vi "buildquery.vi"(1 "String":string="status") -> (0 "JSON字符串":string)   [LabVIEW 2017]
panel:
  in  "输入簇":cluster{"command":string, "item":string}
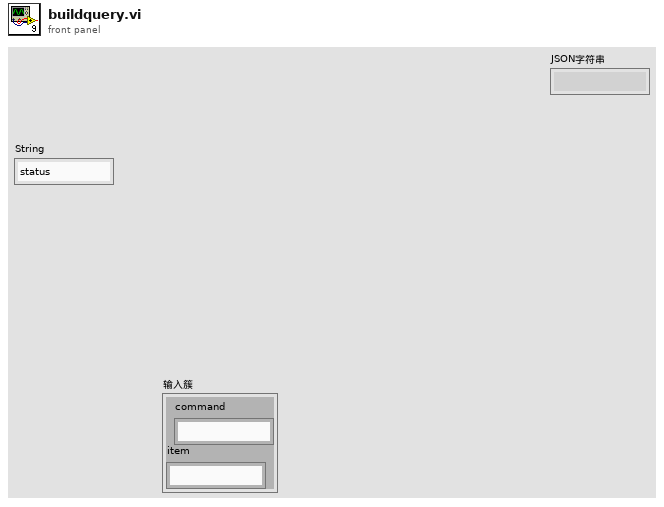
[diagram p1: front panel]
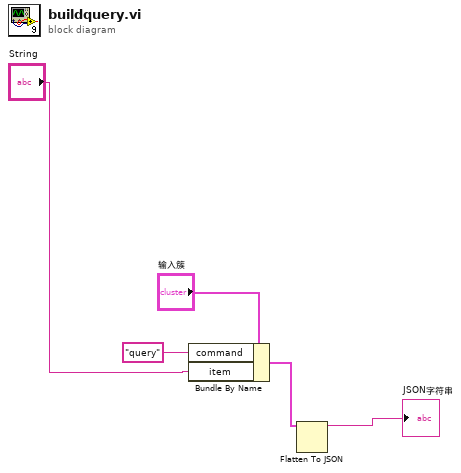
[diagram p0: block diagram]
diagram:
  n1 = Bundle By Name(cluster="输入簇", "command"="query", "item"="String") -> (w3:cluster{"command":string, "item":string})
  n2 = Flatten To JSON(anything=w3) -> (JSON string=→"JSON字符串":string)  [unwired: 2 in, 1 out]
